vi "Package Directory.vi"(11 "Destination Path":path) -> (3 "String":string)   [LabVIEW 2015]
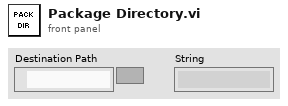
[diagram p1: front panel]
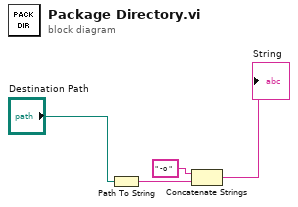
[diagram p0: block diagram]
diagram:
  n1 = Path To String(path="Destination Path") -> (string=w3:string)
  n2 = Concatenate Strings(" -o " ("string"), w3) -> (→"String":string)
